vi "Write Key (Double).vi"(4 "format (fractional)":T2(ring), 5 "use system decimal point (T)":bool=TRUE, 6 "precision (6)":i16=6, 7 "section":string, 8 "error in (no error)":errorcluster, 9 "value":dbl, 10 "key":string, 11 "refnum":T1) -> (0 "error out":errorcluster, 2 "found?":bool, 3 "refnum out":T1)   [LabVIEW 2020, in "NI_LVConfig.lvlib"]
doc: "Writes a value to a key in a specified section of the configuration data identified by <B>refnum</B>. This VI modifies data in memory. To write data to disk, use the Close Config Data VI. Wire data to the <B>value</B> input to determine the polymorphic instance to use or manually select the instance."
uses:
  NI_LVConfig.lvlib
  Config Data RefNum.ctl
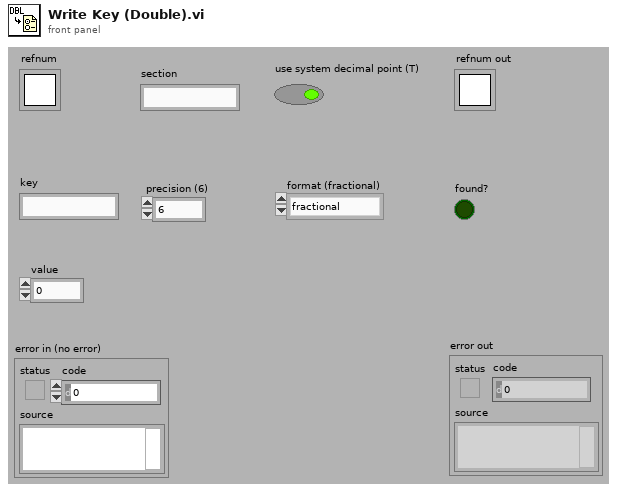
[diagram p1: front panel]
types:
  T1 = typedef "NI_LVConfig.lvlib/Config Data RefNum.ctl" = refnum<k1>
  T2 = enum16{"fractional", "engineering", "exponential"}
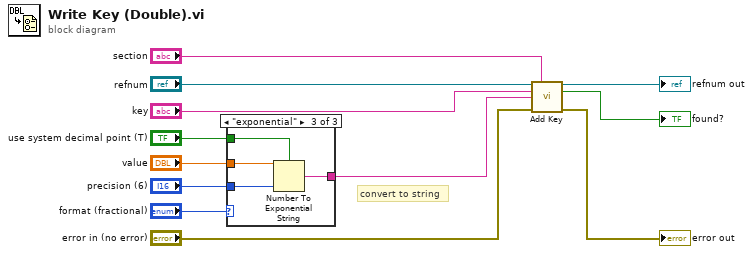
[diagram p0: block diagram]
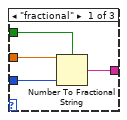
[diagram p2: hidden frame]
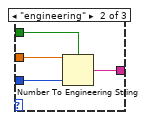
[diagram p3: hidden frame]
diagram:
  # "convert to string"
  n1 = case shown="\"exponential\"" "format (fractional)" {
    tunnel: [w16 w20 w24] -> w1
    tunnel: "precision (6)" -> [w14 w19 w21]
    tunnel: "value" -> [w15 w18 w22]
    tunnel: "use system decimal point (T)" -> [w13 w17 w23]
    frame "fractional" {
      n2 = Number To Fractional String(use system decimal point (T)=w13, number=w15, precision (6)=w14) -> (F-format string=w16:string)  [unwired: 1 out]
    }
    frame "engineering" {
      n3 = Number To Engineering String(1:w17, 2:w19, 4:w18) -> (0:w20:string)  [unwired: 1 out]
    }
    frame "exponential" {
      n4 = Number To Exponential String(number=w22, precision (6)=w21, 1:w23) -> (E-format string=w24:string)  [unwired: 1 out]
    }
  }
  n5 = call "Add Key.vi"("refnum"="refnum", "section"="section", "key"="key", "value"=w1, "error in (no error)"="error in (no error)") -> ("refnum out"=→"refnum out":T1, "key exists?"=→"found?":bool, "error out"=→"error out":errorcluster)  [unwired: 1 in, 7 out]
